vi "CRYSet Channel Table Front Panel.vi"(11 "Vi Ref":refnum<vi>) -> ()   [LabVIEW 2013]
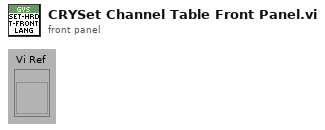
[diagram p1: front panel]
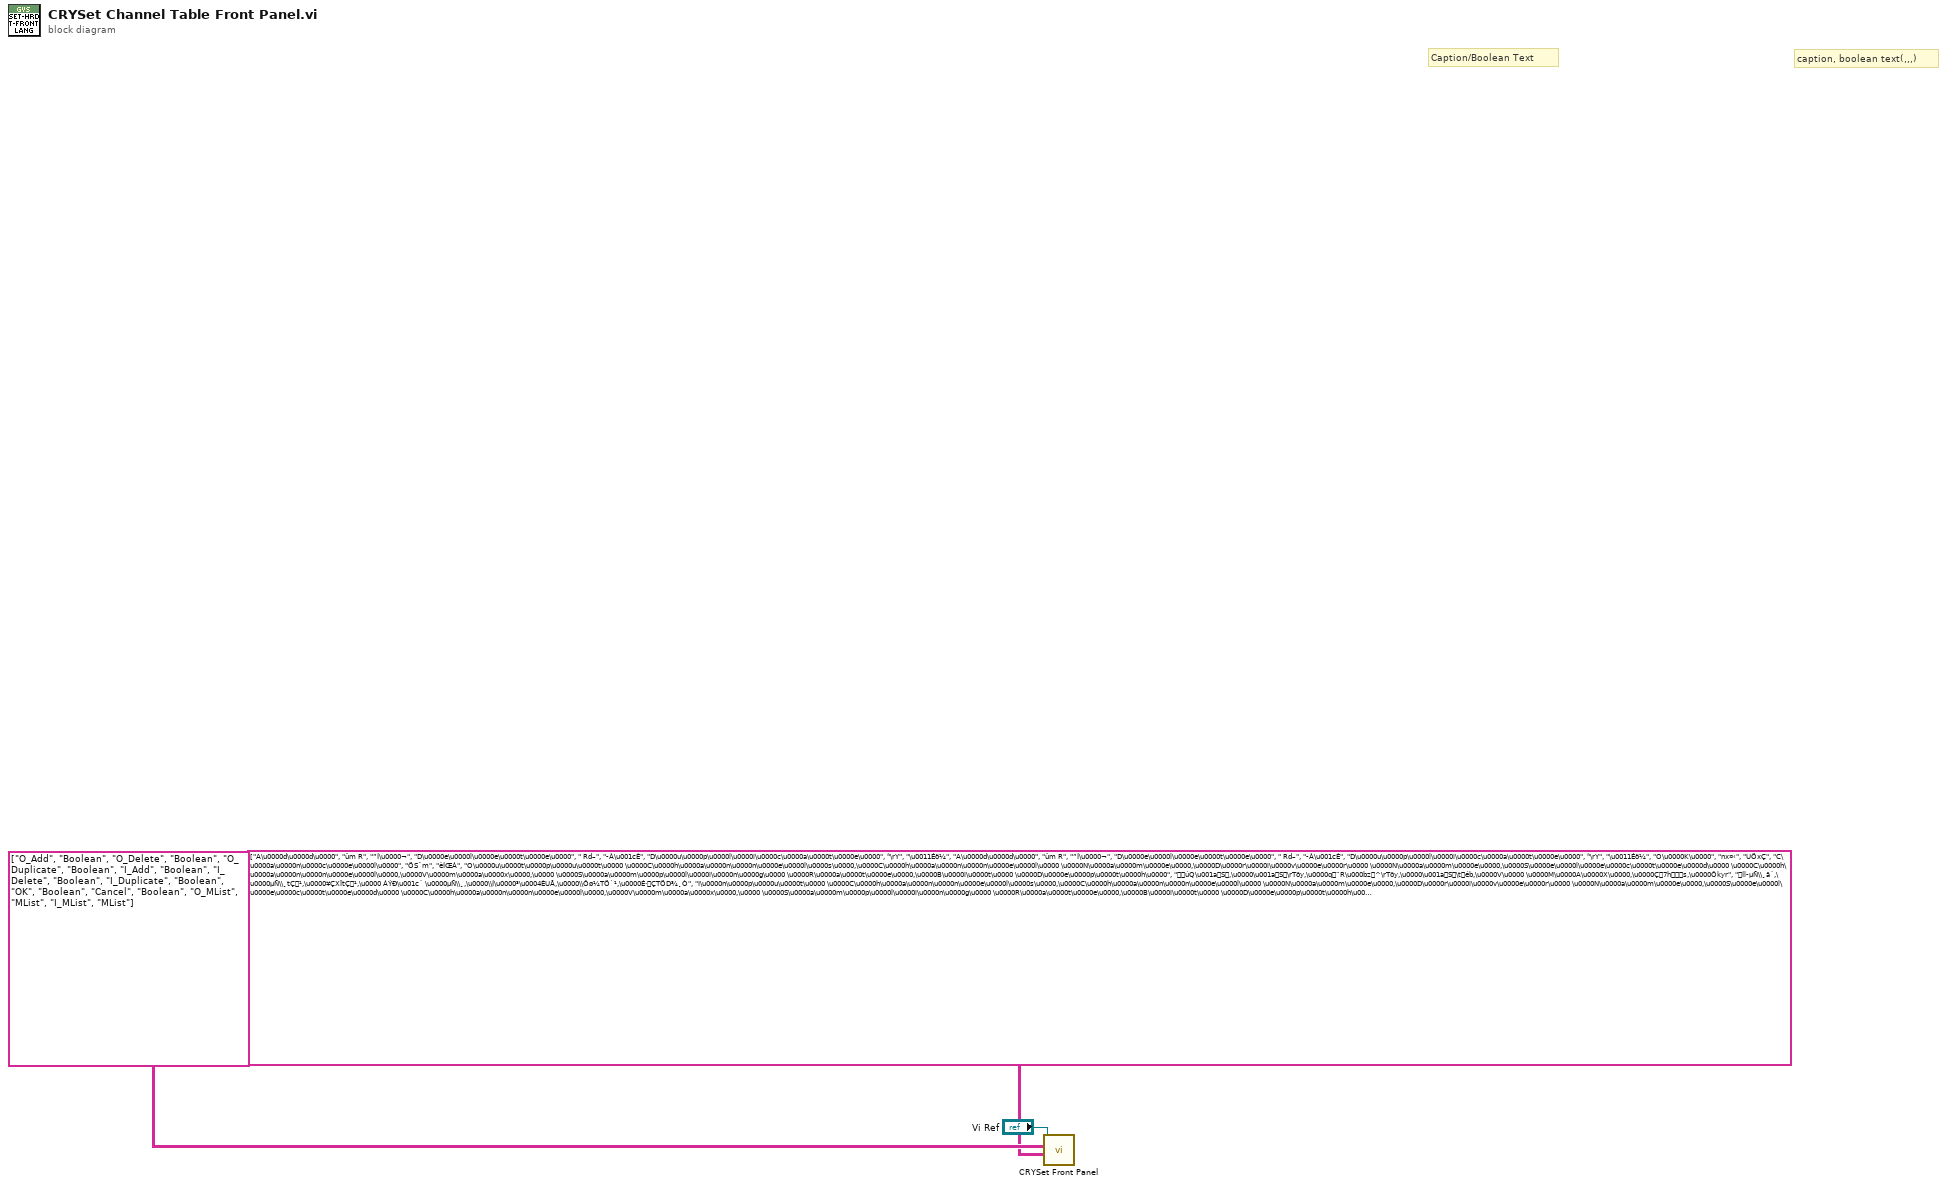
[diagram p0: block diagram]
diagram:
  # "caption, boolean text(,,,)"
  # "Caption/Boolean Text"
  n1 = call "CRYSet Front Panel.vi"("Caption(Boolean Text)"=string[][] [["A\u0000d\u0000d\u0000", "ûm R", "”Í\u0000¬"], ["D\u0000e\u0000l\u0000e\u0000t\u0000e\u0000", " Rd–", "­À\u001cÈ"], ["D\u0000u\u0000p\u0000l\u0000i\u0000c\u0000a\u0000t\u0000e\u0000", "͑\rY", "\u0011Éõ¼"], ["A\u0000d\u0000d\u0000", "ûm R", "”Í\u0000¬"], ["D\u0000e\u0000l\u0000e\u0000t\u0000e\u0000", " Rd–", "­À\u001cÈ"], ["D\u0000u\u0000p\u0000l\u0000i\u0000c\u0000a\u0000t\u0000e\u0000", "͑\rY", "\u0011Éõ¼"], ["O\u0000K\u0000", "nx¤‹", "UÖxÇ"], ["C\u0000a\u0000n\u0000c\u0000e\u0000l\u0000", "ÖSˆm", "èÍŒÁ"], ["O\u0000u\u0000t\u0000p\u0000u\u0000t\u0000 \u0000C\u0000h\u0000a\u0000n\u0000n\u0000e\u0000l\u0000s\u0000,\u0000C\u0000h\u0000a\u0000n\u0000n\u0000e\u0000l\u0000 \u0000N\u0000a\u0000m\u0000e\u0000,\u0000D\u0000r\u0000i\u0000v\u0000e\u0000r\u0000 \u0000N\u0000a\u0000m\u0000e\u0000,\u0000S\u0000e\u0000l\u0000e\u0000c\u0000t\u0000e\u0000d\u0000 \u0000C\u0000h\u0000a\u0000n\u0000n\u0000e\u0000l\u0000,\u0000V\u0000m\u0000a\u0000x\u0000,\u0000 \u0000S\u0000a\u0000m\u0000p\u0000l\u0000i\u0000n\u0000g\u0000 \u0000R\u0000a\u0000t\u0000e\u0000,\u0000B\u0000i\u0000t\u0000 \u0000D\u0000e\u0000p\u0000t\u0000h\u0000", "úQ\u001aS,\u0000\u001aS\rTðy,\u0000q¨R\u000bz^\rTðy,\u0000\u001aS\téb,\u0000V\u0000 \u0000M\u0000A\u0000X\u0000,\u0000Ç7hs,\u0000Ôkyr", "Íl­µÑ\\¸ä´,\u0000µÑ\\¸tÇ¹,\u0000¥ÇXÎtÇ¹,\u0000 ÁÝÐ\u001c´ \u0000µÑ\\¸,\u0000\\Í\u0000³\u0004ÈUÅ,\u0000\\Ôø¼TÖ`¹,\u0000É·ÇTÖD¾¸Ò"], ["I\u0000n\u0000p\u0000u\u0000t\u0000 \u0000C\u0000h\u0000a\u0000n\u0000n\u0000e\u0000l\u0000s\u0000,\u0000C\u0000h\u0000a\u0000n\u0000n\u0000e\u0000l\u0000 \u0000N\u0000a\u0000m\u0000e\u0000,\u0000D\u0000r\u0000i\u0000v\u0000e\u0000r\u0000 \u0000N\u0000a\u0000m\u0000e\u0000,\u0000S\u0000e\u0000l\u0000e\u0000c\u0000t\u0000e\u0000d\u0000 \u0000C\u0000h\u0000a\u0000n\u0000n\u0000e\u0000l\u0000,\u0000V\u0000m\u0000a\u0000x\u0000,\u0000 \u0000S\u0000a\u0000m\u0000p\u0000l\u0000i\u0000n\u0000g\u0000 \u0000R\u0000a\u0000t\u0000e\u0000,\u0000B\u0000i\u0000t\u0000 \u0000D\u0000e\u0000p\u0000t\u0000h\u0000,\u0000L\u0000a\u0000t\u0000e\u0000n\u0000c\u0000y\u0000", "eQ\u001aS,\u0000\u001aS\rTðy,\u0000q¨R\u000bz^\rTðy,\u0000\u001aS\téb,\u0000V\u0000 \u0000M\u0000A\u0000X\u0000,\u0000Ç7hs,\u0000Ôkyr,\u0000ö^ß", "Çl­µÑ\\¸ä´,\u0000µÑ\\¸tÇ¹,\u0000¥ÇXÎtÇ¹,\u0000 ÁÝÐ\u001c´ \u0000µÑ\\¸,\u0000\\Í\u0000³\u0004ÈUÅ,\u0000\\Ôø¼TÖ`¹,\u0000É·ÇTÖD¾¸Ò,\u0000ÀÉðÅ"]], "Control ID and Type(Label Name, Type)"=string[][] [["O_Add", "Boolean"], ["O_Delete", "Boolean"], ["O_Duplicate", "Boolean"], ["I_Add", "Boolean"], ["I_Delete", "Boolean"], ["I_Duplicate", "Boolean"], ["OK", "Boolean"], ["Cancel", "Boolean"], ["O_MList", "MList"], ["I_MList", "MList"]], "Vi Ref"="Vi Ref") -> ()  [unwired: 9 in]
